vi "load_hyst_sat_parallel_data.vi"() -> (0 "Hyst[U_nom]":dbl[](array[numeric]), 1 "U_nom":dbl[](array[numeric]), 3 "input cluster":T1)   [LabVIEW 2017, in "Sat_Hyst_TestCase.lvclass"]
uses:
  Sat_Hyst_TestCase.lvclass
  <vilib>/Utility/file.llb/Read Delimited Spreadsheet (DBL).vi
panel:
  in  "input cluster 2":T1
  out "N_sat":i32
  out "TF-order":i32
  out "wp":dbl[](array[numeric])
  out "rp":dbl[](array[numeric])
  out "wsp":dbl[](array[numeric])
  out "dp":dbl[](array[numeric])
  out "den":dbl[](array[numeric])
  out "num":dbl[](array[numeric])
  out "N_hyst":i32
  out "all rows":dbl[][](array[numeric])
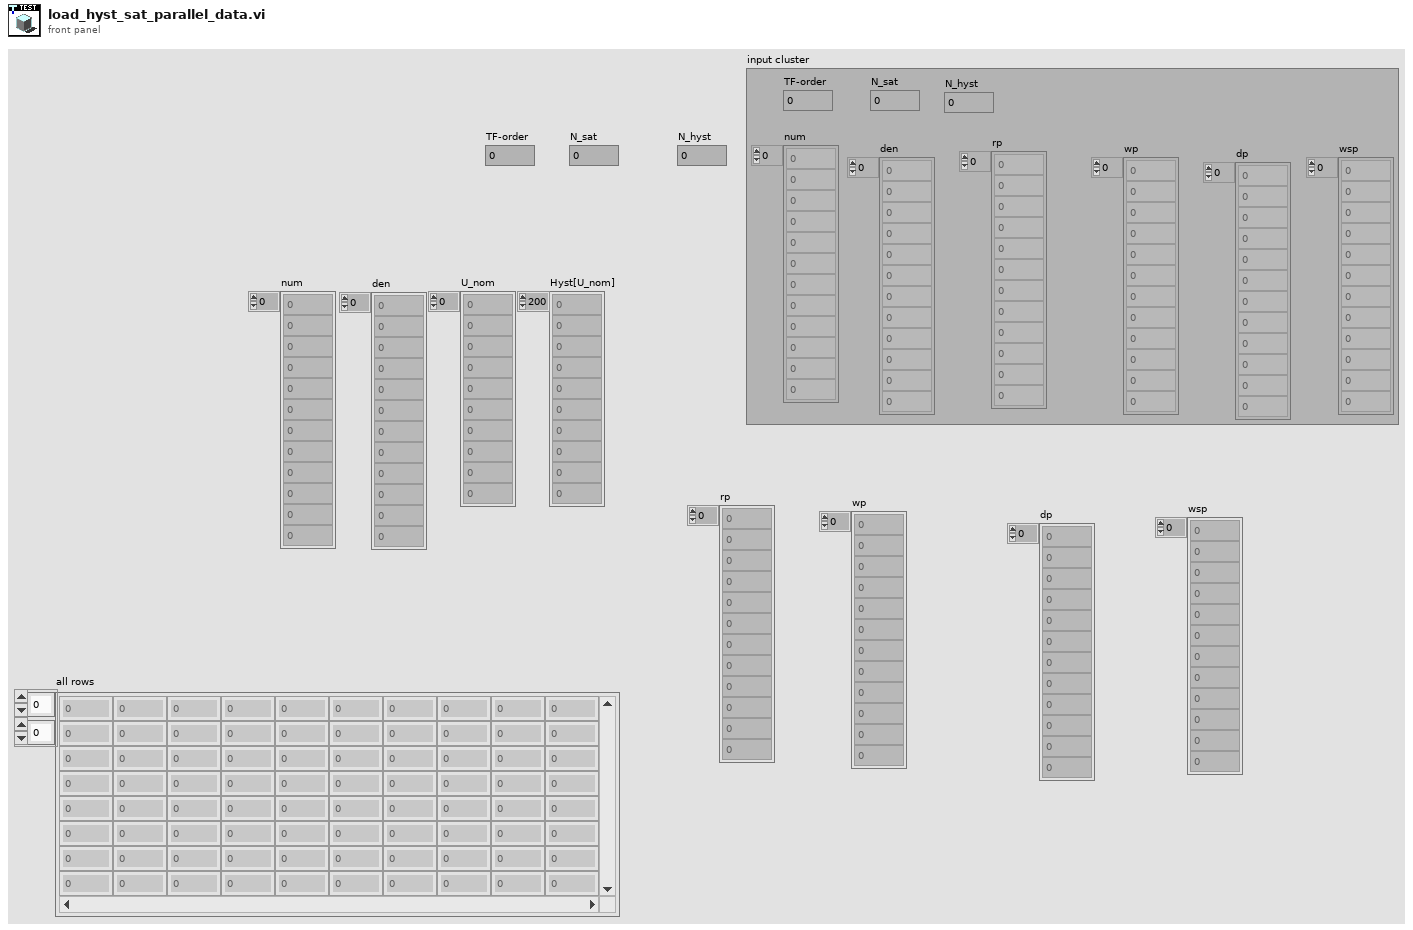
[diagram p1: front panel]
types:
  T1 = cluster{"TF-order":i32, "N_sat":i32, "N_hyst":i32, "num":dbl[], "wsp":dbl[], "dp":dbl[], "rp":dbl[], "wp":dbl[], "den":dbl[]}
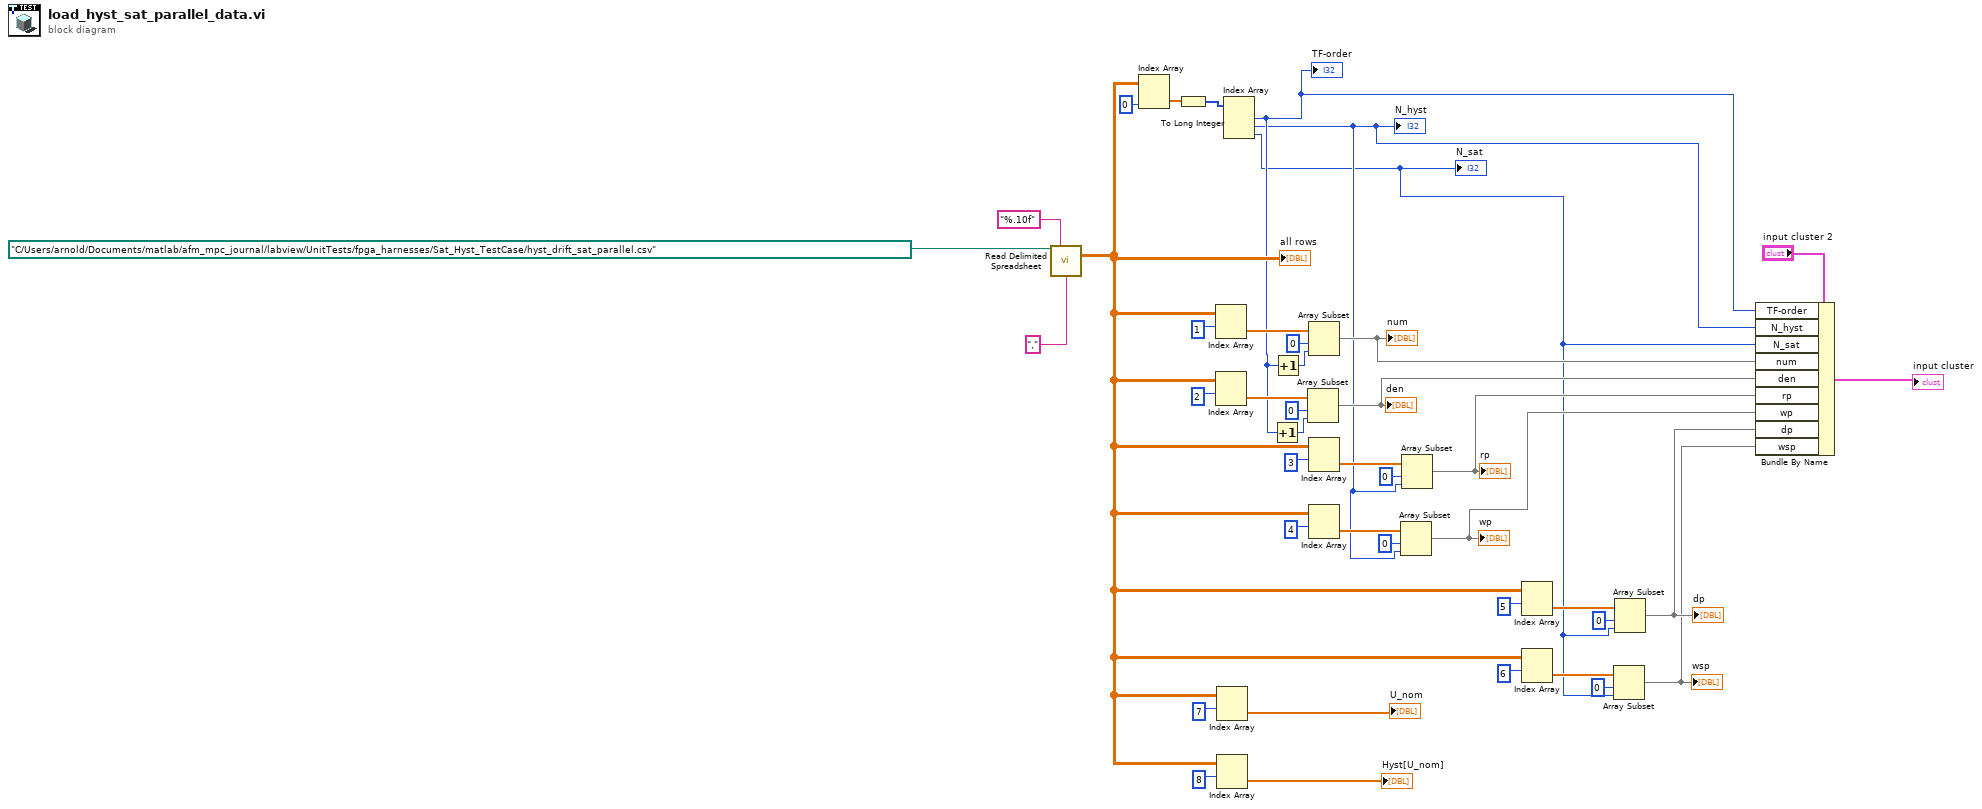
[diagram p0: block diagram]
diagram:
  n1 = call-poly <vilib>:"Read Delimited Spreadsheet.vi"("file path (dialog if empty)"=path "C:/Users/arnold/Documents/matlab/afm_mpc_journal/labview/UnitTests/fpga_harnesses/Sat_Hyst_TestCase/hyst_drift_sat_parallel.csv" ("Path"), "format (%.3f)"="%.10f", "delimiter (\\t)"="," ("delimiter (\\t)")) -> ("all rows"=w14:dbl[][])  [unwired: 7 in, 5 out]
  "all rows" <- w14
  n2 = Index Array(array=w14, index (row)=0) -> (element=w33:dbl[])  [unwired: 1 in]
  n3 = To Long Integer(number=w33) -> (32bit integer=w15:i32[])
  n4 = Index Array(array=w14, index (row)=1) -> (element=w38:dbl[])  [unwired: 1 in]
  n5 = Index Array(array=w14, index (row)=2) -> (element=w35:dbl[])  [unwired: 1 in]
  n6 = Index Array(array=w14, index (row)=7) -> (element=→"U_nom":dbl[])  [unwired: 1 in]
  n7 = Index Array(array=w14, index (row)=8) -> (element=→"Hyst[U_nom]":dbl[])  [unwired: 1 in]
  n8 = Index Array(array=w15) -> (element #1=w5:i32, element #2=w4:i32, element #3=w3:i32)  [unwired: 3 in]
  "N_hyst" <- w4
  "TF-order" <- w5
  "N_sat" <- w3
  n9 = Increment(x=w5) -> (x+1=w12:i32)
  n10 = Increment(x=w5) -> (x+1=w13:i32)
  n11 = Array Subset(array=w35, index=0, length=w12) -> (w10:dbl[])
  "den" <- w10
  n12 = Array Subset(array=w38, index=0, length=w13) -> (w11:dbl[])
  "num" <- w11
  n13 = Index Array(array=w14, index (row)=3) -> (element=w20:dbl[])  [unwired: 1 in]
  n14 = Index Array(array=w14, index (row)=4) -> (element=w17:dbl[])  [unwired: 1 in]
  n15 = Array Subset(array=w17, index=0, length=w4) -> (w8:dbl[])
  "wp" <- w8
  n16 = Array Subset(array=w20, index=0, length=w4) -> (w9:dbl[])
  "rp" <- w9
  n17 = Index Array(array=w14, index (row)=5) -> (element=w26:dbl[])  [unwired: 1 in]
  n18 = Index Array(array=w14, index (row)=6) -> (element=w23:dbl[])  [unwired: 1 in]
  n19 = Array Subset(array=w23, index=0, length=w3) -> (w6:dbl[])
  "wsp" <- w6
  n20 = Array Subset(array=w26, index=0, length=w3) -> (w7:dbl[])
  "dp" <- w7
  n21 = Bundle By Name(cluster="input cluster 2", "TF-order"=w5, "N_hyst"=w4, "N_sat"=w3, "num"=w11, "den"=w10, "rp"=w9, "wp"=w8, "dp"=w7, "wsp"=w6) -> (→"input cluster":T1)
